vi "Configure Start Trigger [STT].vi"(7 "Trigger Slope (Positive)":i32(ring) caption="trigger slope (Positive)" items=["Positive", "Negative", "Either"], 8 "error in (no error)":errorcluster, 9 "Trigger Source (None)":string(combo) caption="trigger source (None)", 10 "Channel Name (\"\")":string="CHANNEL1" caption="channel name (\"CHANNEL1\")", 11 "CS++Fgen in":refnum<class "CS++Fgen.lvclass">) -> (0 "error out":errorcluster, 3 "CS++Fgen out":refnum<class "CS++Fgen.lvclass">)   [LabVIEW 2016, in "CS++Fgen.lvlib" / "CS++Fgen.lvclass"]
doc: "This VI configures the properties that control the function generator's start trigger. These properties are the start trigger source and slope.\n\nA start trigger initiates generation of a waveform or sequence. \n\nNote:\n\n(1) This VI is part of the IviFgenStartTrigger [STT] extension group."
uses:
  CS++Fgen.lvclass
  CSPP_Core/Classes/CS++ProcessVariables/ProcessVariable/PV.lvclass
  PV-Enum-n.ctl
  CSPP_Core/Classes/CS++ProcessVariables/ProcessVariable/PV.lvclass/PV.ctl
  CS++Fgen.lvclass/CS++Fgen.ctl
  CSPP_Core/Classes/CS++ProcessVariables/ProcessVariable/Write Data.vi
  CSPP_Core/Classes/CS++ProcessVariables/ProcessVariable/Write Timestamp.vi
  CSPP_Core/Classes/CS++ProcessVariables/ProcessVariable/Write Quality.vi
  CSPP_Core/Classes/CS++ProcessVariables/ProcessVariable/Write status.vi
  CSPP_Core/Classes/CS++ProcessVariables/PVConnection/PVConnection.lvclass
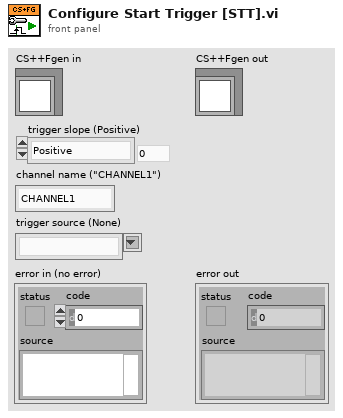
[diagram p1: front panel]
types:
  T1 = typedef "CS++Fgen.lvlib/CS++Fgen.lvclass/PV-Enum-n.ctl" = enum16{"Amplitude", "Arb-Frequency", "DCOffset", "Frequency", "OutputImpedance", "StartPhase", "AdvancedTriggerSlope", "AM-Source", "BurstCount", "FM-Source", "OperationMode", "ResumeTriggerSlope", "StartTriggerSlope", "StopTriggerSlope", "Waveform", "TriggerSource", "AM-Enabled", "ChannelEnabled", "FM-Enabled", "AdvancedTriggerSource", "ResumeTriggerSource", "StartTriggerSource", "StopTriggerSource"}
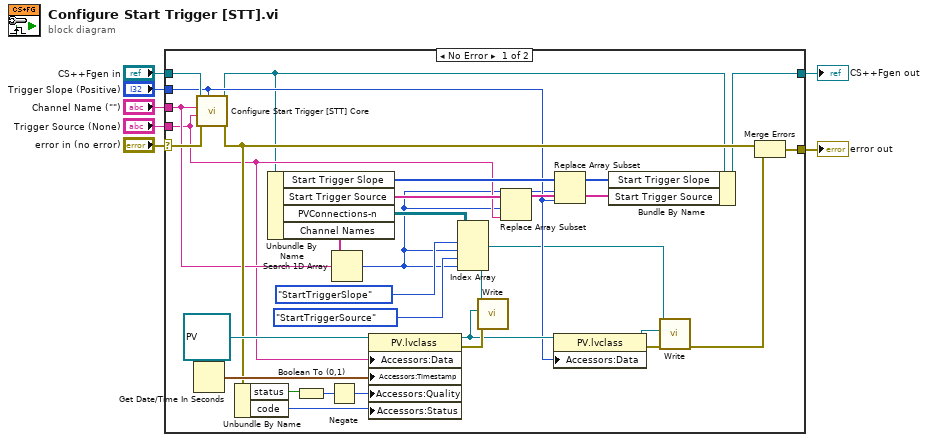
[diagram p0: block diagram]
diagram:
  n1 = case shown="No Error" "error in (no error)" {
    selector: "error in (no error)" -> [w37 w40]
    tunnel: [w14 w40] -> w6
    tunnel: [w12 w39] -> w4
    tunnel: "CS++Fgen in" -> [w38 w39]
    tunnel: "Trigger Slope (Positive)" -> [w15 _]
    tunnel: "Channel Name (\"\")" -> [w17 _]
    tunnel: "Trigger Source (None)" -> [w16 _]
    frame No Error {
      n2 = Get Date/Time In Seconds() -> (seconds since 1Jan1904=w36:timestamp)
      n3 = call-dynamic "Configure Start Trigger [STT] Core.vi"("Trigger Slope (Positive)"=w15, "error in (no error)"=w37, "Trigger Source (None)"=w16, "Channel Name (\"\")"=w17, "CS++Fgen in"=w38) -> ("error out"=w18:errorcluster, "CS++Fgen out"=w13:refnum<class "CS++Fgen.lvclass">)  [unwired: 5 in]
      n4 = Unbundle By Name(w18) -> ("status"=w30:bool, "code"=w28:i32)
      n5 = Unbundle By Name(w13) -> ("Start Trigger Slope"=w24:i32[], "Start Trigger Source"=w26:string[], "PVConnections-n"=w32:refnum<class "PVConnection.lvclass">[][], "Channel Names"=w33:string[])
      n6 = Boolean To (0,1)(Boolean=w30) -> (0, 1=w29:i16)
      n7 = Negate(x=w29) -> (-x=w27:i16)
      n8 = Search 1D Array(1D array=w33, element=w17) -> (index of element=w8:i32)  [unwired: 1 in]
      n9 = property class="PV.lvclass"(reference=refnum<class "PV.lvclass"> refnum ("PV"), "Accessors:Data"=w16, "Accessors:Timestamp"=w36, "Accessors:Quality"=w27, "Accessors:Status"=w28) -> (reference out=w20:refnum<class "PV.lvclass">, error out=w34:errorcluster)  [unwired: 1 in]
      n10 = Index Array(array=w32, index (row) #1=PV-Enum-n."StartTriggerSlope" ("PV-Enum-n"), index (col) #1=w8, index (row) #2=PV-Enum-n."StartTriggerSource" ("PV-Enum-n"), index (col) #2=w8) -> (element #1=w10:refnum<class "PVConnection.lvclass">, element #2=w31:refnum<class "PVConnection.lvclass">)
      n11 = call "Write.vi"("error in (no error)"=w34, "PV"=w20, "PVConnection in"=w31) -> ()  [unwired: 7 in, 2 out]
      n12 = Replace Array Subset(array=w26, new element=w16, index=w8) -> (w25:string[])
      n13 = property class="PV.lvclass"(reference=w20, "Accessors:Data"=w15) -> (reference out=w22:refnum<class "PV.lvclass">, error out=w21:errorcluster)  [unwired: 1 in]
      n14 = Replace Array Subset(array=w24, new element=w15, index=w8) -> (w23:i32[])
      n15 = Bundle By Name(cluster=w13, "Start Trigger Slope"=w23, "Start Trigger Source"=w25) -> (w12:refnum<class "CS++Fgen.lvclass">)
      n16 = call "Write.vi"("error in (no error)"=w21, "PV"=w22, "PVConnection in"=w10) -> ("error out"=w19:errorcluster)  [unwired: 7 in, 1 out]
      n17 = Merge Errors(w18, w19) -> (w14:errorcluster)
    }
    frame Error {
    }
  }
  "error out" <- w6
  "CS++Fgen out" <- w4
